vi "SVL Measure Signal Delay.vi"(0 "reference signal":waveform(dbl), 1 "delayed signal":waveform(dbl), 2 "method":u16(ring)=1 items=["Trigger", "Cross correlation", "Phase lag"], 3 "ignore time stamp":bool=TRUE, 5 "error in (no error)":errorcluster, 7 "trigger parameters":T1={"slope"=1, "level"=0.0, "hysteresis"=-0.1} {"slope" items=["Falling Edge", "Rising Edge"]}) -> (14 "signal delay [samples]":dbl=nan, 19 "error out":errorcluster)   [LabVIEW 2017, in "SoundVib_Transient.lvlib"]
uses:
  <vilib>/addons/Sound and Vibration/svt_Transients/SoundVib_Transient.lvlib
  <vilib>/Analysis/baseanly.llb/Mean (DBL).vi
  <vilib>/measure/matone.llb/Extract Single Tone Information 1 Chan.vi
  <vilib>/Analysis/2dsp.llb/1D Cross Correlation (DBL).vi
  <vilib>/measure/mamon.llb/Trigger Detection for 1 Channel.vi
  <vilib>/Analysis/NI_AALPro.lvlib
  <vilib>/measure/NI_MAPro.lvlib
  <vilib>/Analysis/NI_AAL_SigProc.lvlib
  <vilib>/Analysis/NI_AALBase.lvlib
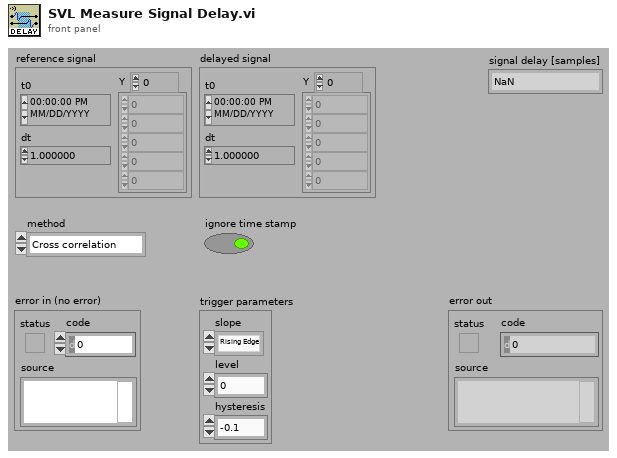
[diagram p1: front panel]
types:
  T1 = cluster{"slope":u16, "level":dbl, "hysteresis":dbl}
  T2 = cluster{"approx freq. (optional)":dbl, "search (+/- % of Fsampl.)":dbl}
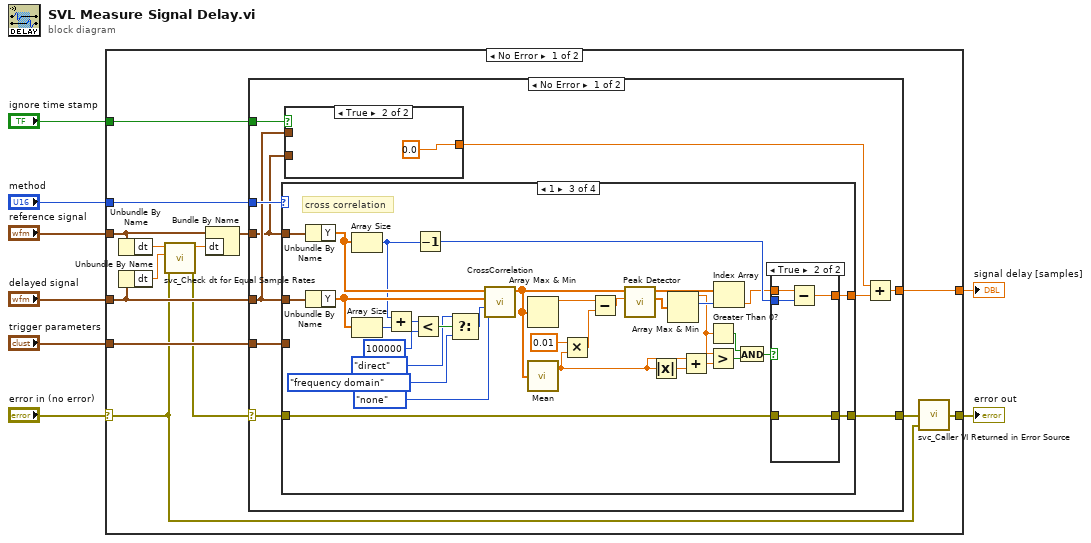
[diagram p0: block diagram]
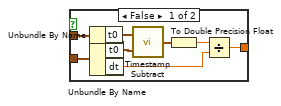
[diagram p2: hidden frame]
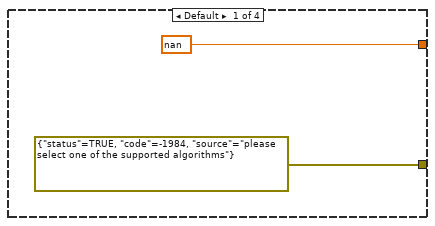
[diagram p3: hidden frame]
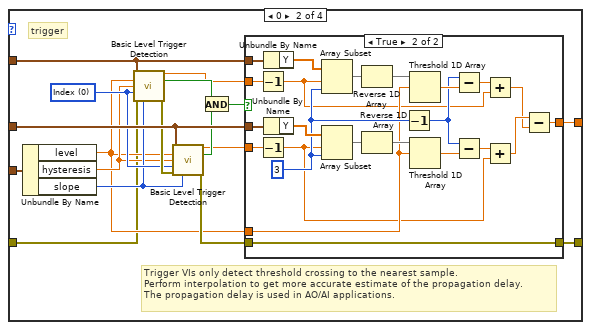
[diagram p4: hidden frame]
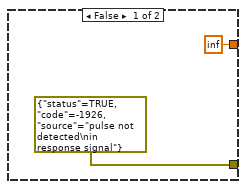
[diagram p5: hidden frame]
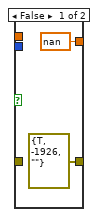
[diagram p6: hidden frame]
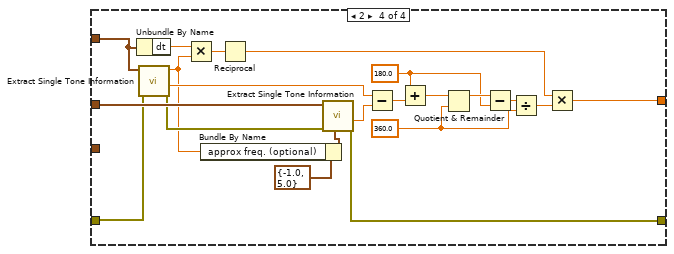
[diagram p7: hidden frame]
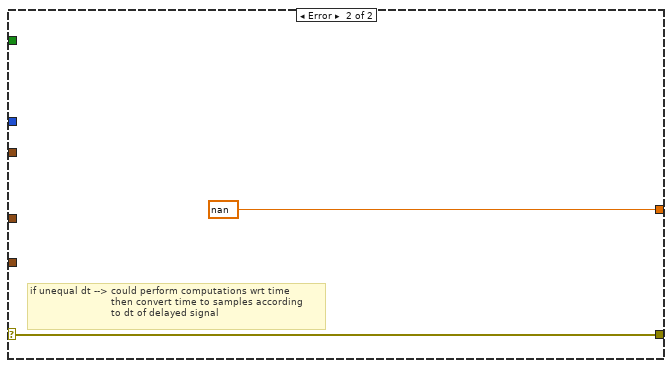
[diagram p8: hidden frame]
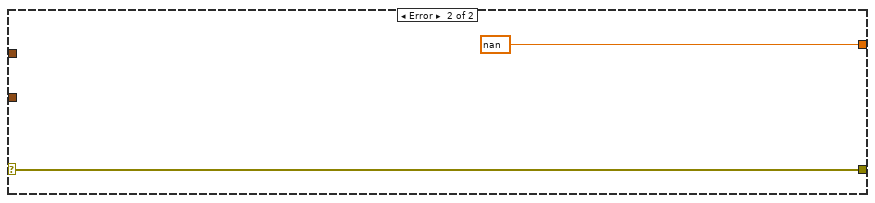
[diagram p9: hidden frame]
diagram:
  n1 = case shown="No Error" "error in (no error)" {
    selector: "error in (no error)" -> [w13 w148]
    tunnel: "method" -> [w22 _]
    tunnel: "trigger parameters" -> [w21 _]
    tunnel: [w14 w148] -> w6
    tunnel: "delayed signal" -> [w17 _]
    tunnel: "reference signal" -> [w11 _]
    tunnel: "ignore time stamp" -> [w19 _]
    tunnel: [w18 nan] -> w2
    frame No Error {
      n2 = Unbundle By Name(w11) -> ("dt"=w16:dbl)
      n3 = Unbundle By Name(w17) -> ("dt"=w15:dbl)
      n4 = call <vilib>:"svc_Check dt for Equal Sample Rates.vi"("error in (no error)"=w13, "dt Y"=w15, "dt X"=w16) -> ("error out"=w12:errorcluster, "dt Y"=w9:dbl)  [unwired: 7 in]
      n5 = Bundle By Name(cluster=w11, "dt"=w9) -> (w10:waveform(dbl))
      n6 = case shown="No Error" w12 {
        selector: w12 -> [w24 w147]
        tunnel: w22 -> [w32 _]
        tunnel: w21 -> [w31 _]
        tunnel: [w30 w147] -> w20
        tunnel: w19 -> [w29 _]
        tunnel: [w28 nan] -> w18
        tunnel: w17 -> [w25 _]
        tunnel: w10 -> [w23 _]
        frame No Error {
          n7 = case shown="1" w32 {
            tunnel: w25 -> [_ w60 w96 w145]
            tunnel: w23 -> [_ w59 w98 w138]
            tunnel: [nan w58 w115 w133] -> w27
            tunnel: w31 -> [_ w49 _ _]
            tunnel: w24 -> [_ w45 w99 w144]
            tunnel: [errorcluster {"status"=TRUE, "code"=-1984, "source"="please select one of the supported algorithms"} ("error out") w44 w113 w129] -> w30
            frame Default {
            }
            frame 0 {
              w50 = u16 0 items=["Index", "Time"] ("mode")
              # "trigger"
              # "Trigger VIs only detect threshold crossing to the nearest sample. \nPerform interpolation to get more accurate estimate of the propagation delay.\nThe propagation delay is used in AO/AI applications."
              n8 = Unbundle By Name(w49) -> ("level"=w46:dbl, "hysteresis"=w47:dbl, "slope"=w48:u16)
              n9 = call-poly <vilib>:"Basic Level Trigger Detection.vi"("signal in"=w59, "level"=w46, "hysteresis"=w47, "location mode"=w50, "error in (no error)"=w45, "trigger slope"=w48) -> ("trigger location"=w52:dbl, "trigger detected?"=w57:bool, "error out"=w55:errorcluster)  [unwired: 7 in]
              n10 = call-poly <vilib>:"Basic Level Trigger Detection.vi"("signal in"=w60, "level"=w46, "hysteresis"=w47, "location mode"=w50, "error in (no error)"=w55, "trigger slope"=w48) -> ("trigger location"=w53:dbl, "trigger detected?"=w56:bool, "error out"=w54:errorcluster)  [unwired: 7 in]
              n11 = And(x=w57, y=w56) -> (x .and. y?=w51:bool)
              n12 = case shown="True" w51 {
                tunnel: w53 -> [_ w70]
                tunnel: w52 -> [_ w82]
                tunnel: [inf w85] -> w58
                tunnel: w54 -> [_ w84]
                tunnel: [errorcluster {"status"=TRUE, "code"=-1926, "source"="pulse not detected\nin response signal"} ("error out") w84] -> w44
                tunnel: w59 -> [_ w83]
                tunnel: w46 -> [_ w69]
                tunnel: w60 -> [_ w74]
                frame False {
                }
                frame True {
                  w71 = 3 ("length")
                  n13 = Decrement(x=w82) -> (x-1=w66:dbl)
                  n14 = Decrement(x=w70) -> (x-1=w65:dbl)
                  n15 = Unbundle By Name(w83) -> ("Y"=w81:dbl[])
                  n16 = Unbundle By Name(w74) -> ("Y"=w73:dbl[])
                  n17 = Array Subset(array=w81, index=w66, length=w71) -> (w80:dbl[])
                  n18 = Array Subset(array=w73, index=w65, length=w71) -> (w75:dbl[])
                  n19 = Reverse 1D Array(array=w80) -> (reversed array=w79:dbl[])
                  n20 = Reverse 1D Array(array=w75) -> (reversed array=w76:dbl[])
                  n21 = Decrement(x=w71) -> (x-1=w72:i32)
                  n22 = Threshold 1D Array(2:w69, 3:w79) -> (0:w78:dbl)  [unwired: 1 in]
                  n23 = Threshold 1D Array(2:w69, 3:w76) -> (0:w77:dbl)  [unwired: 1 in]
                  n24 = Subtract(x=w72, y=w78) -> (x-y=w67:dbl)
                  n25 = Subtract(x=w72, y=w77) -> (x-y=w68:dbl)
                  n26 = Add(x=w67, y=w66) -> (x+y=w63:dbl)
                  n27 = Add(x=w68, y=w65) -> (x+y=w64:dbl)
                  n28 = Subtract(x=w64, y=w63) -> (x-y=w85:dbl)
                }
              }
            }
            frame 1 {
              # "cross correlation"
              n29 = Unbundle By Name(w98) -> ("Y"=w97:dbl[])
              n30 = Unbundle By Name(w96) -> ("Y"=w95:dbl[])
              n31 = Array Size(array=w97) -> (size(s)=w94:i32)
              n32 = Array Size(array=w95) -> (size(s)=w93:i32)
              n33 = Add(x=w94, y=w93) -> (x+y=w92:i32)
              n34 = Less?(x=w92, y=100000) -> (x < y?=w90:bool)
              n35 = Decrement(x=w94) -> (x-1=w114:i32)
              n36 = Select(t=enum32{"direct", "frequency domain"}."direct" ("algorithm"), s=w90, f=enum32{"direct", "frequency domain"}."frequency domain" ("algorithm")) -> (s? t:f=w87:enum32{"direct", "frequency domain"})
              n37 = call-poly <vilib>:"CrossCorrelation.vi"("normalization"=enum32{"none", "unbiased", "biased"}."none", "algorithm"=w87, "Y"=w95, "X"=w97) -> ("Rxy"=w109:dbl[])  [unwired: 6 in, 1 out]
              n38 = Array Max & Min(array=w109) -> (max value=w118:dbl)  [unwired: 3 out]
              n39 = call-poly <vilib>:"Mean.vi"("X"=w109) -> ("mean"=w102:dbl)  [unwired: 1 out]
              n40 = Multiply(x=0.01, y=w102) -> (x*y=w101:dbl)
              n41 = Subtract(x=w118, y=w101) -> (x-y=w117:dbl)
              n42 = call <vilib>:"Peak Detector.vi"("threshold"=w117, "X"=w109) -> ("Amplitudes"=w116:dbl[], "Locations"=w112:dbl[])  [unwired: 5 in, 3 out]
              n43 = Absolute Value(x=w102) -> (abs(x)=w107:dbl)
              n44 = Array Max & Min(array=w116) -> (max value=w104:dbl, max index (indices)=w111:i32)  [unwired: 2 out]
              n45 = Add(x=w102, y=w107) -> (x+y=w108:dbl)
              n46 = Greater Than 0?(x=w104) -> (x > 0?=w103:bool)
              n47 = Greater?(x=w104, y=w108) -> (0:w105:bool)
              n48 = Index Array(array=w112, index=w111) -> (element=w110:dbl)
              n49 = And(x=w103, y=w105) -> (x .and. y?=w106:bool)
              n50 = case shown="True" w106 {
                tunnel: [nan w124] -> w115
                tunnel: w114 -> [_ w123]
                tunnel: w99 -> [_ w122]
                tunnel: [errorcluster {"status"=TRUE, "code"=-1926, "source"=""} ("error out") w122] -> w113
                tunnel: w110 -> [_ w121]
                frame False {
                }
                frame True {
                  n51 = Subtract(x=w121, y=w123) -> (x-y=w124:dbl)
                }
              }
            }
            frame 2 {
              w125 = 180.0 ("y")
              w131 = 360.0 ("y")
              n52 = Unbundle By Name(w138) -> ("dt"=w137:dbl)
              n53 = call-poly <vilib>:"Extract Single Tone Information.vi"("error in (no error)"=w144, "time signal in"=w138) -> ("error out"=w143:errorcluster, "detected phase (deg)"=w140:dbl, "detected frequency"=w136:dbl)  [unwired: 4 in, 3 out]
              n54 = Multiply(x=w137, y=w136) -> (x*y=w134:dbl)
              n55 = Bundle By Name(cluster=T2 {"approx freq. (optional)"=-1.0, "search (+/- % of Fsampl.)"=5.0} ("advanced search"), "approx freq. (optional)"=w136) -> (w141:T2)
              n56 = Reciprocal(x=w134) -> (1/x=w130:dbl)
              n57 = call-poly <vilib>:"Extract Single Tone Information.vi"("advanced search"=w141, "error in (no error)"=w143, "time signal in"=w145) -> ("error out"=w129:errorcluster, "detected phase (deg)"=w139:dbl)  [unwired: 3 in, 4 out]
              n58 = Subtract(x=w140, y=w139) -> (x-y=w126:dbl)
              n59 = Add(x=w125, y=w126) -> (x+y=w128:dbl)
              n60 = Quotient & Remainder(x=w128, y=w131) -> (x-y*floor(x/y)=w135:dbl)  [unwired: 1 out]
              n61 = Subtract(x=w135, y=w125) -> (x-y=w127:dbl)
              n62 = Divide(x=w127, y=w131) -> (x/y=w132:dbl)
              n63 = Multiply(x=w130, y=w132) -> (x*y=w133:dbl)
            }
          }
          n64 = case shown="True" w29 {
            tunnel: w25 -> [w40 _]
            tunnel: w23 -> [w39 _]
            tunnel: [w34 0.0] -> w26
            frame False {
              n65 = Unbundle By Name(w40) -> ("t0"=w38:timestamp)
              n66 = Unbundle By Name(w39) -> ("t0"=w37:timestamp, "dt"=w33:dbl)
              n67 = call <vilib>:"Timestamp Subtract.vi"("y"=w37, "x"=w38) -> ("x - y"=w36:timestamp)
              n68 = To Double Precision Float(number=w36) -> (double precision float=w35:dbl)
              n69 = Divide(x=w35, y=w33) -> (x/y=w34:dbl)
            }
            frame True {
            }
          }
          n70 = Add(x=w26, y=w27) -> (x+y=w28:dbl)
        }
        frame Error {
          # "if unequal dt --> could perform computations wrt time \n                           then convert time to samples according\n                           to dt of delayed signal"
        }
      }
      n71 = call <vilib>:"svc_Caller VI Returned in Error Source.vi"("warning input to caller"=w13, "error in (no error)"=w20) -> ("error out"=w14:errorcluster)  [unwired: 3 in]
    }
    frame Error {
    }
  }
  "signal delay [samples]" <- w2
  "error out" <- w6
